vi "Add Tx Status Section.vi"(8 "error in":errorcluster, 11 "Custom Device Ref in":T1 format="%.0x") -> (0 "error out":errorcluster, 1 "Tx Status channel Refs":T1[](array[typedef]) format="%.0x", 2 "Tx Status Section Ref out":T1 format="%.0x", 3 "Custom Device Ref out":T1 format="%.0x")   [LabVIEW 2020, in "afdx_custom_device Scripting.lvlib"]
uses:
  afdx_custom_device Scripting.lvlib
  <vilib>/NI VeriStand/Custom Device API/Custom Device Item Ref.ctl
  <vilib>/NI VeriStand/Custom Device API/Custom Device Channel.ctl
  <vilib>/NI VeriStand/Custom Device API/Custom Device Channel Type.ctl
  Constants.vi
  <vilib>/NI VeriStand/Custom Device API/Custom Device API.lvlib
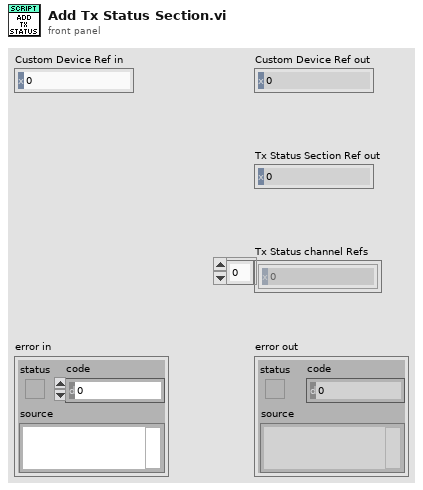
[diagram p1: front panel]
types:
  T1 = typedef "Custom Device API.lvlib/Custom Device Item Ref.ctl" = u64
  T2 = typedef "Custom Device API.lvlib/Custom Device Channel.ctl" = cluster{"Type":T3, "Units":string, "Default Value":dbl, "Faultable":bool, "Scalable":bool}
  T3 = typedef "Custom Device API.lvlib/Custom Device Channel Type.ctl" = enum16{"Input", "Output"}
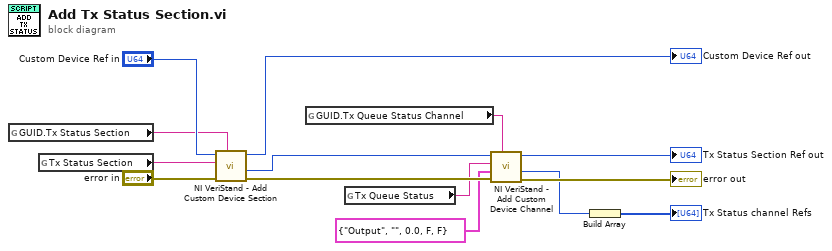
[diagram p0: block diagram]
diagram:
  n1 = global read "Constants.vi" "GUID.Tx Status Section"() -> (w10:string)
  n2 = global read "Constants.vi" "Tx Status Section"() -> (w12:string)
  n3 = call <vilib>:"NI VeriStand - Add Custom Device Section.vi"("GUID (Default Section)"=w10, "error in (no error)"="error in", "Section Name"=w12, "Parent Ref in"="Custom Device Ref in") -> ("error out"=w11:errorcluster, "Section Ptr"=w6:T1, "Parent Ref out"=→"Custom Device Ref out":T1)  [unwired: 4 in, 1 out]
  n4 = global read "Constants.vi" "GUID.Tx Queue Status Channel"() -> (w8:string)
  n5 = global read "Constants.vi" "Tx Queue Status"() -> (w9:string)
  n6 = call <vilib>:"NI VeriStand - Add Custom Device Channel.vi"("GUID (Default Channel)"=w8, "error in (no error)"=w11, "Channel"=T2 {"Type"=enum."Output", "Units"="", "Default Value"=0.0, "Faultable"=FALSE, "Scalable"=FALSE}, "Channel Name"=w9, "Parent Ref in"=w6) -> ("error out"=→"error out":errorcluster, "Channel Ref"=w3:T1, "Parent Ref out"=→"Tx Status Section Ref out":T1)  [unwired: 3 in, 1 out]
  n7 = Build Array(w3) -> (→"Tx Status channel Refs":T1[])
